vi "Sub Routing program.vi"(5 "Image":refnum<vi>, 6 "Test Name":refnum<vi>, 7 "FeedBack Channel":string[](array[string]), 8 "error in (no error)":errorcluster, 9 "Feature Step Enable":T1(array[cluster]), 10 "Table":refnum<vi>, 11 "queue Out in":refnum<queue>) -> (0 "error out":errorcluster, 1 "Error":bool, 2 "reference out":refnum<vi>, 3 "Queue out":refnum<queue>)   [LabVIEW 2015]
uses:
  Test  enqueue/AutoTest seq.ctl
  Galobal variable_TI.vi
panel:
  out "2D Picture 2":picture
  out "error out 2":errorcluster
  out "2D Picture":picture
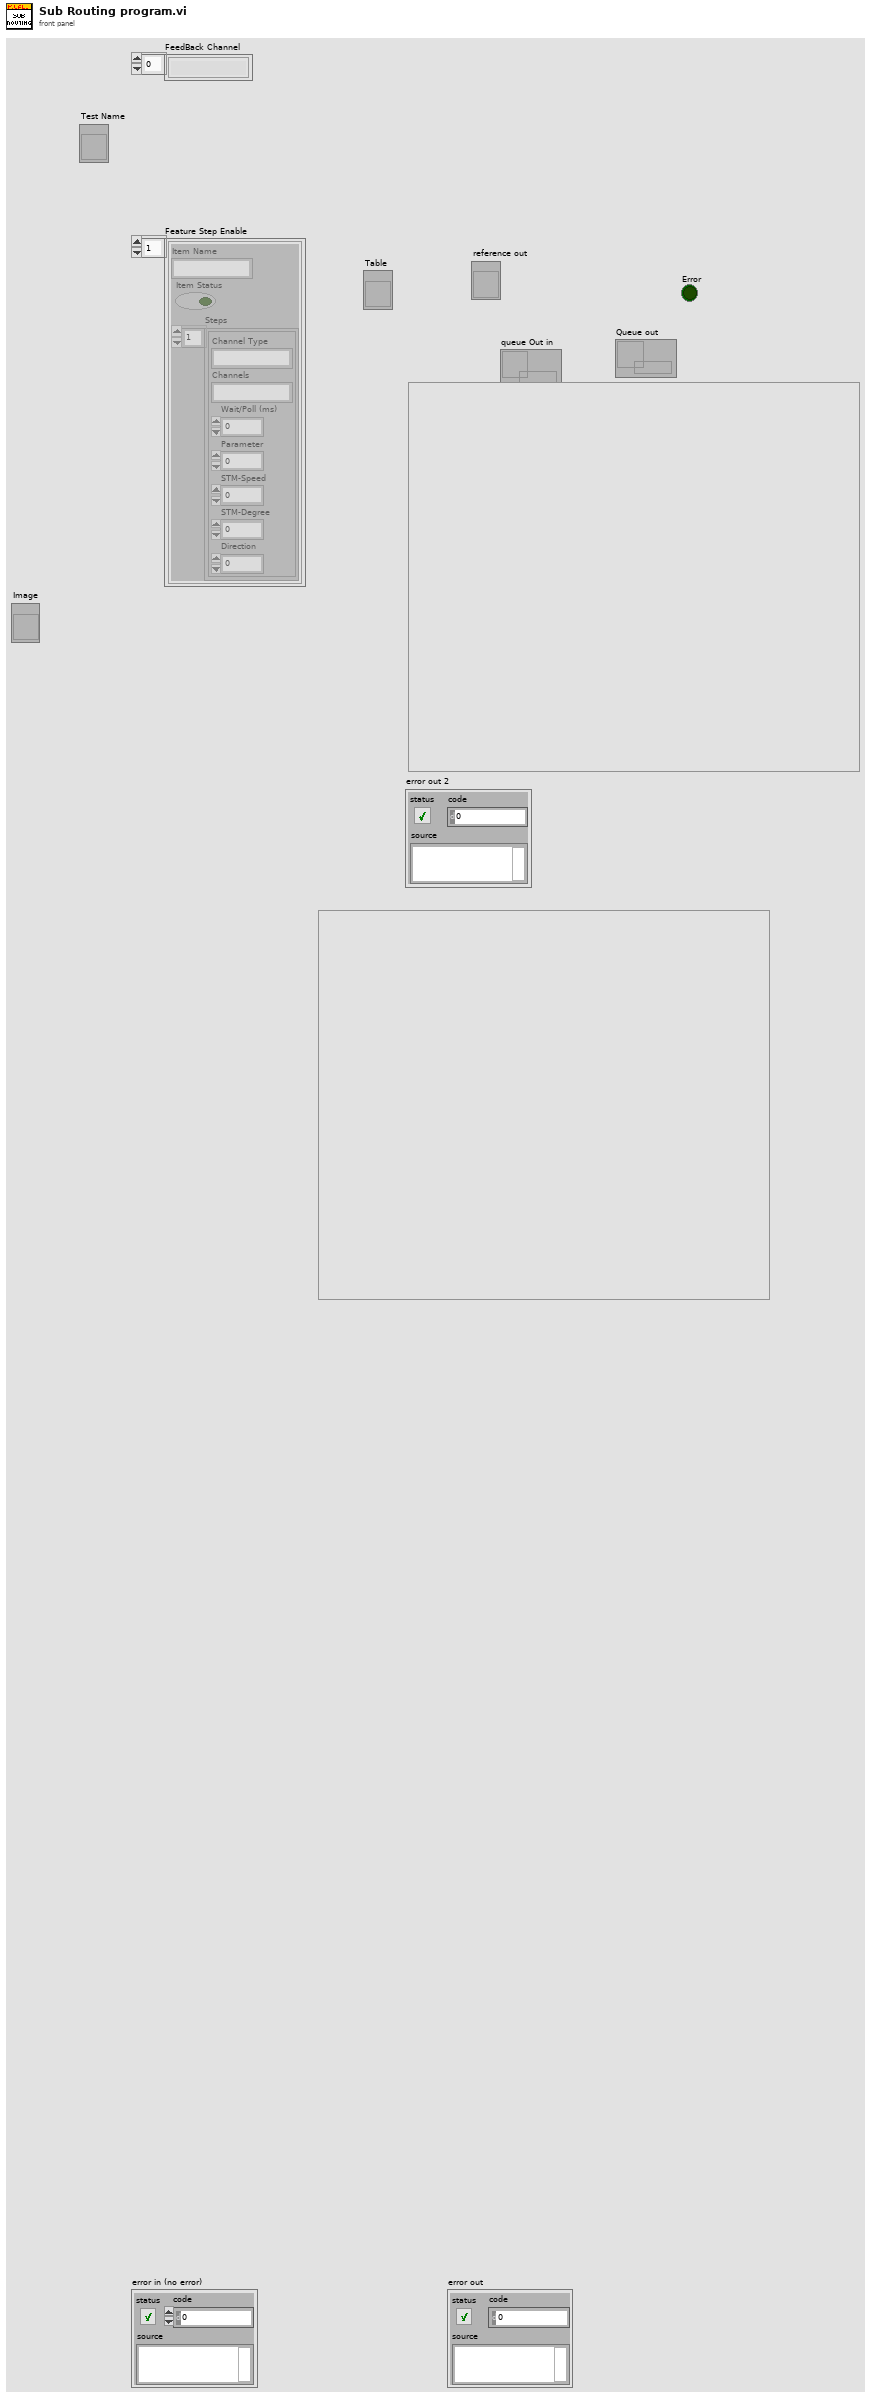
[diagram p1: front panel]
types:
  T1 = cluster{"Item Name":string, "Item Status":bool, "Steps":cluster{"Channel Type":string, "Channels":string, "Wait/Poll (ms)":u32, "Parameter":u8, "STM-Speed":i32, "STM-Degree":u32, "Direction":u8}[]}[]
  T2 = cluster{"Zoom Factor":sgl, "Horizontal position":sgl, "Vertical position":sgl}[]
  T3 = cluster{"Channel Type":string, "Channels":string, "Wait/Poll (ms)":u32, "Parameter":u8, "STM-Speed":i32, "STM-Degree":u32, "Direction":u8}[]
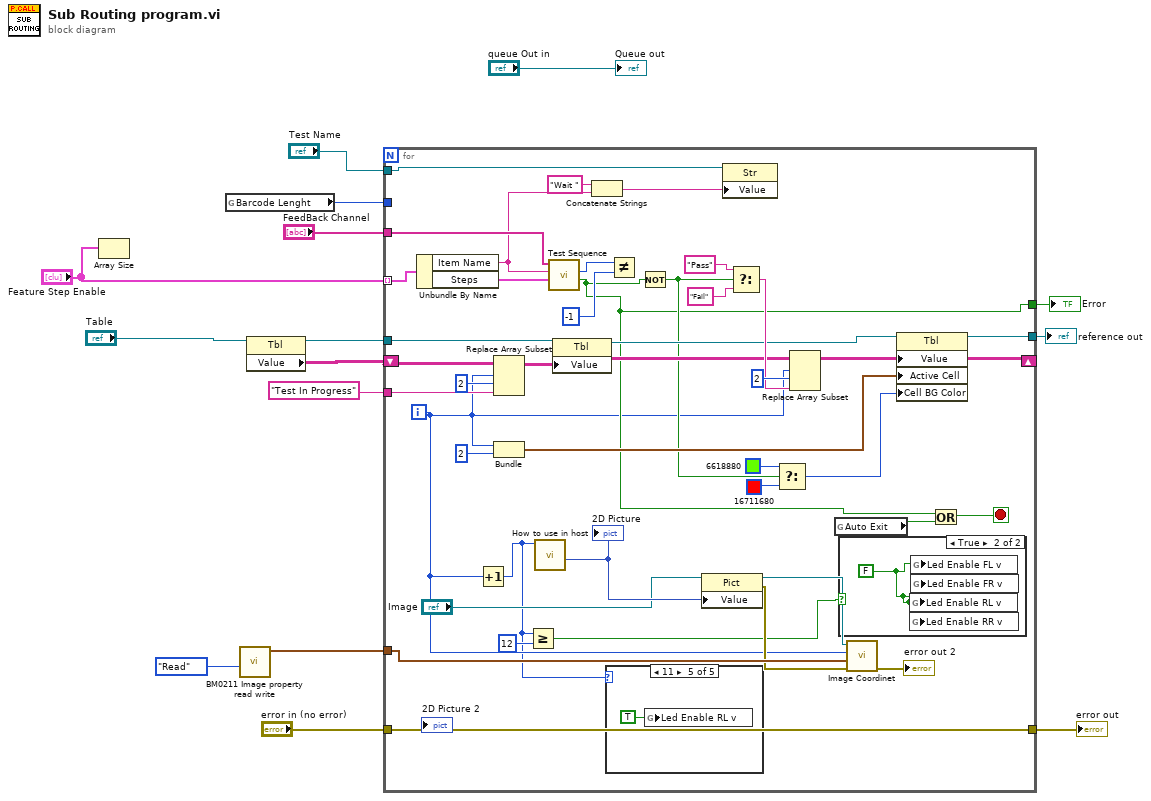
[diagram p0: block diagram]
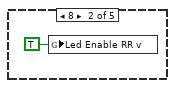
[diagram p3: hidden frame]
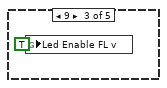
[diagram p4: hidden frame]
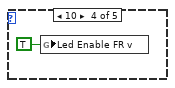
[diagram p5: hidden frame]
diagram:
  n1 = Array Size(array="Feature Step Enable") -> ()  [unwired: 1 out]
  n2 = global read "Galobal variable_TI.vi" "Barcode Lenght"() -> (w14:i32)
  n3 = call "BM0211 Image property read write.vi"("Read write"=enum16{"write", "Read"}."Read") -> ("Out"=w1:T2)  [unwired: 9 in, 1 out]
  n4 = property class="Tbl"(reference="Table") -> (reference out=w8:refnum<vi>, "Value"=w11:string[][])  [unwired: 1 in, 1 out]
  n5 = for {
    tunnel: "Feature Step Enable" -> [w56] mode=indexing
    tunnel: "FeedBack Channel" -> [w53]
    tunnel: w14 -> [_]
    shift-right: [w37] -> _
    shift-left: w11 -> [w49]
    tunnel: "Test In Progress" ("new element/subarray") -> [w48]
    tunnel: w8 -> [w47]
    tunnel: [w38] -> w7
    tunnel: "error in (no error)" -> [w36]
    tunnel: [w36] -> w5
    tunnel: [w31] -> w4
    tunnel: "Test Name" -> [w30]
    tunnel: w1 -> [w25]
    i -> [w19]
    stop <- w23 stop-if-true
    n6 = Unbundle By Name(w56) -> ("Item Name"=w28:string, "Steps"=w52:T3)
    n7 = Increment(x=w19) -> (x+1=w16:i32)
    n8 = Replace Array Subset(array=w49, new element=w48, index (row)=w19, index (col)=2 ("disabled index (col)")) -> (w44:string[][])
    n9 = Bundle(w19, 2) -> (w43:cluster{i32, i32})  [unwired: 1 in]
    n10 = Greater Or Equal?(x=w16, y=12) -> (x >= y?=w17:bool)
    n11 = call "How to use in host.vi"("Select Part"=w16) -> ("2D Picture"=w26:picture)  [unwired: 10 in]
    "2D Picture" <- w26
    n12 = call "Test Sequence.vi"("FeedBack Channel"=w53, "Test Name"=w28, "Steps"=w52) -> ("Out"=w35:i32, "Condition"=w31:bool)  [unwired: 4 in, 1 out]
    n13 = property class="Tbl"(reference=w47, "Value"=w44) -> (reference out=w39:refnum<vi>)  [unwired: 1 in, 1 out]
    n14 = Concatenate Strings("Wait " ("string"), w28) -> (w27:string)
    n15 = case shown="11" w16 {
      frame 0, Default {
      }
      frame 8 {
        n16 = global write "Galobal variable_TI.vi" "Led Enable RR v"(TRUE ("Led Enable RR v")) -> ()
      }
      frame 9 {
        n17 = global write "Galobal variable_TI.vi" "Led Enable FL v"(TRUE ("Led Enable FL v")) -> ()
      }
      frame 10 {
        n18 = global write "Galobal variable_TI.vi" "Led Enable FR v"(TRUE ("Led Enable FR v")) -> ()
      }
      frame 11 {
        n19 = global write "Galobal variable_TI.vi" "Led Enable RL v"(TRUE ("Led Enable RL v")) -> ()
      }
    }
    n20 = Not Equal?(x=w35, y=-1) -> ()  [unwired: 1 out]
    n21 = Not(x=w31) -> (.not. x?=w32:bool)
    n22 = property class="Pict"(reference="Image", "Value"=w26) -> (reference out=w22:refnum<vi>, error out=w21:errorcluster)  [unwired: 1 in]
    n23 = property class="Str"(reference=w30, "Value"=w27) -> ()  [unwired: 1 in, 2 out]
    n24 = Select(t="Pass", s=w32, f="Fail") -> (s? t:f=w45:string)
    n25 = Select(t=u32 6618880 ("Color Box"), s=w32, f=u32 16711680 ("Color Box")) -> (s? t:f=w40:u32)
    n26 = Replace Array Subset(array=w44, new element=w45, index (row)=w19, index (col)=2 ("disabled index (col)")) -> (w37:string[][])
    n27 = global read "Galobal variable_TI.vi" "Auto Exit"() -> (w33:bool)
    n28 = case shown="True" w17 {
      frame False {
      }
      frame True {
        w61 = FALSE
        n29 = global write "Galobal variable_TI.vi" "Led Enable RL v"(w61) -> ()
        n30 = global write "Galobal variable_TI.vi" "Led Enable RR v"(w61) -> ()
        n31 = global write "Galobal variable_TI.vi" "Led Enable FL v"(w61) -> ()
        n32 = global write "Galobal variable_TI.vi" "Led Enable FR v"(w61) -> ()
      }
    }
    n33 = call "Image Coordinet.vi"("error in (no error)"=w21, "Out"=w25, "index of element"=w19, "Picture in"=w22) -> ("error out"=→"error out 2":errorcluster)  [unwired: 7 in]
    n34 = property class="Tbl"(reference=w39, "Value"=w37, "Active Cell"=w43, "Cell BG Color"=w40) -> (reference out=w38:refnum<vi>)  [unwired: 1 in, 1 out]
    n35 = Or(x=w31, y=w33) -> (x .or. y?=w23:bool)
  }
  "error out" <- w5
  "reference out" <- w7
  "Error" <- w4
  "Queue out" <- "queue Out in"
